vi "Graphics-Draw Hexagon.vi"(0 "X":dbl, 5 "Width":dbl=1.0, 7 "Y":dbl, 9 "Height":dbl=1.0, 11 "Ramp":dbl) -> (8 "X-Y graph":cluster{dbl[], dbl[]})   [LabVIEW 2015]
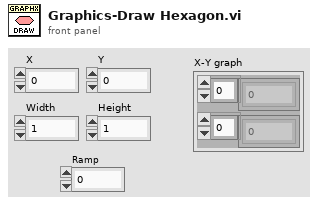
[diagram p1: front panel]
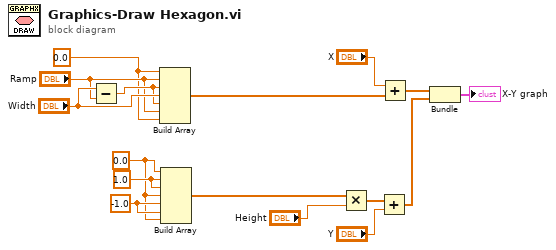
[diagram p0: block diagram]
diagram:
  w1 = 0.0
  w4 = 0.0
  w2 = 1.0
  w16 = -1.0
  n1 = Subtract(x="Width", y="Ramp") -> (x-y=w6:dbl)
  n2 = Build Array(w4, "Ramp", w6, "Width", w6, "Ramp", w4) -> (w3:dbl[])
  n3 = Build Array(w1, w2, w2, w1, w16, w16, w1) -> (w14:dbl[])
  n4 = Multiply(x=w14, y="Height") -> (x*y=w13:dbl[])
  n5 = Add(x=w13, y="Y") -> (x+y=w12:dbl[])
  n6 = Add(x="X", y=w3) -> (x+y=w15:dbl[])
  n7 = Bundle(w15, w12) -> (→"X-Y graph":cluster{dbl[], dbl[]})  [unwired: 1 in]
